vi "Stop Engine.vi"(8 "Error In":errorcluster, 11 "LQCoreEngine":refnum<class "LQCoreEngine.lvclass">) -> (0 "Error Out":errorcluster)   [LabVIEW 2013, in "Template.lvlib" / "LQCoreEngine.lvclass"]
uses:
  LQCoreEngine.lvclass
  _Private/Global Quit Event Holder.vi
  Template.lvlib
panel:
  # "Copyright (c) 2016 Sze Howe Koh\n\nThis Source Code Form is subject to the terms of the Mozilla Public\nLicense, v. 2.0. If a copy of the MPL was not distributed with this\nfile, You can obtain one at http://mozilla.org/MPL/2.0/."
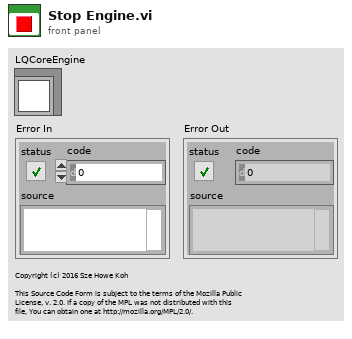
[diagram p1: front panel]
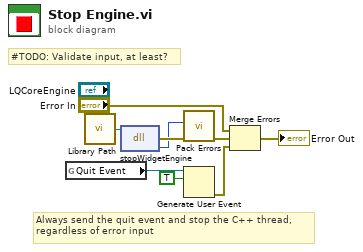
[diagram p0: block diagram]
diagram:
  # "#TODO: Validate input, at least?"
  # "Always send the quit event and stop the C++ thread,\nregardless of error input"
  n1 = global read "Global Quit Event Holder.vi" "Quit Event"() -> (w9:refnum<user-event>)
  n2 = call "Library Path.vi"() -> ("Library Path"=w7:path)
  n3 = dll-call lib="?" fn="stopWidgetEngine"(path in=w7) -> (error out=w6:errorcluster, "errorCode"=w5:i32)  [unwired: 2 in, 1 out]
  n4 = call "Pack Errors.vi"("Error In"=w6, "Error Code"=w5) -> ("Error Out"=w4:errorcluster)  [unwired: 9 in]
  n5 = Generate User Event(user event=w9, event data cluster=TRUE ("event data")) -> (error out=w3:errorcluster)  [unwired: 2 in, 1 out]
  n6 = Merge Errors("Error In", w4, w3) -> (→"Error Out":errorcluster)
